vi "myBOT-Simulate-2DOF-ZV.vi"() -> ()   [LabVIEW 2013]
doc: "\"myBOT-Simulate-2DOF-ZV\": Simulates a myBOT with 2DOF (alpha and gamma) as a state space model. Nonlinear behavior is optional. The myBOT behavior can be simulated with two controller types:\n1) PID-Controller\n2) Model Based Balance Controller\n\nThis VI was created for the myRIO Balancing Robot Project. See https://decibel.ni.com/content/groups/myrio-balancing-robot for more information and example projects."
uses:
  <vilib>/addons/Control Design/_Model Construction/Data Typedefs.llb/CD Variables.ctl
  <vilib>/Simulation/Scripting/Companion Diagram/SimConfigNode/SimParams.ctl
  <vilib>/Simulation/Scripting/Companion Diagram/SimConfigNode/_simSolvers.ctl
  <vilib>/Simulation/Implementation/Shared/SIMSCR Execution Mode.ctl
  <vilib>/Platform/TimedLoop/XDataNode/timing_clust.ctl
  <vilib>/Platform/TimedLoop/XDataNode/nitl_modes.ctl
  <vilib>/Platform/TimedLoop/XDataNode/wakeup.ctl
  <vilib>/Simulation/Param Hierarchy/Typedefs/SIMPH Param Control Actions.ctl
  <vilib>/Simulation/Scripting/Editor Utilities/SIM subVI tag data.ctl
  <vilib>/Simulation/Scripting/Editor Utilities/SIM subVI execution type.ctl
  <vilib>/Simulation/Implementation/Shared/NILVSim_ParamChanged.vi
  <vilib>/Simulation/Implementation/Shared/NILVSim_FinishedLate.vi
  <vilib>/Simulation/Implementation/Shared/NILVSIM_BeginStep.vi
  <vilib>/Simulation/Utility/Implementation/SIM Halt.vi
  <vilib>/Simulation/DataSources/Implementation/NILVSim Pulse Generator.llb/SIM Pulse Generator (scalar).vi
  <vilib>/Simulation/ContinuousLinear/Implementation/NILVSim State Space.llb/SIM State Space Distributor (CD).vi
  <vilib>/Simulation/Nonlinear/Implementation/NILVSim Saturation.llb/SIM Saturation (scalar).vi
  <vilib>/Simulation/Implementation/Shared/SIM Is Init or Final Stage.vi
  <vilib>/Simulation/Nonlinear/Implementation/NILVSim DeadZone.llb/SIM DeadZone (scalar).vi
  <vilib>/Simulation/ContinuousLinear/Implementation/NILVSim State Space.llb/SIM State Space Collector (CD).vi
  <vilib>/Simulation/SignalDisplay/Implementation/NILVSim Time Waveform.llb/SIM Time Waveform (vector).vi
  <vilib>/Simulation/Implementation/Shared/SIM Fire Discrete SubVI.vi
  <vilib>/Simulation/Implementation/Shared/NILVSim_Manager.vi
  <vilib>/Simulation/Implementation/Shared/NILVSim_FinalizeModel.vi
  <vilib>/Simulation/Implementation/Shared/SIM Fire Discrete SubVI (Core).vi
  <vilib>/addons/Control Design/_Model Construction/Model Creation.llb/Model Creation SubVI/cd_Create Symbolic State Space Model.vi
  <vilib>/Simulation/Implementation/Shared/SIM Unbundle Sim Info.vi
  <vilib>/Utility/error.llb/Clear Errors.vi
  <vilib>/Simulation/Implementation/Shared/NILVSim_GetModelError.vi
  <vilib>/Simulation/Implementation/Shared/SIM Bundle Sim Info.vi
  <vilib>/Simulation/Implementation/Shared/SIMSH Read Queue.vi
  <vilib>/Simulation/Implementation/Shared/NILVSim_Initialize.vi
  <vilib>/Simulation/Utility/Implementation/NILVSim Get Time and IsAcceptedStep.vi
  SubVI/myBOT_Draw.vi
  SubVI/myBOT_Nonlinearities.vi
  <vilib>/Simulation/Scripting/Companion Diagram/SimConfigNode/SimDog.xnode
  <vilib>/Simulation/Model Libraries/PID/SIM PID (Parallel).vi
  <vilib>/Simulation/Model Libraries/PID/SIM PID.vi
  <vilib>/Platform/TimedLoop/XDataNode/XDataNode.xnode
  <vilib>/Simulation/Implementation/XNodeFramework/SimXNode/SimX.xnode
  <vilib>/addons/Control Design/_Model Construction/NI_LinSys_Model Creation.lvlib
  <vilib>/addons/Control Design/_Model Construction/Model Typedefs.llb/CD General Elements.ctl
  <vilib>/addons/Control Design/_Model Construction/NI_LinSys_Model Typedefs.lvlib
  <vilib>/addons/Control Design/_Model Construction/Model Typedefs.llb/CD State Space Model (MIMO).ctl
  <vilib>/Simulation/ContinuousLinear/Implementation/NILVSim State Space.llb/SIM State Space (CD).vi
  <vilib>/Platform/TimedLoop/XDataNode/XDNodeRunTimeDep.lvlib
  <vilib>/Simulation/Implementation/Shared/NI_SIM_Implementation.lvlib
  <vilib>/addons/Control Design/_Model Construction/NI_LinSys_Data Typedefs.lvlib
panel:
  in  "Controller:\nBalanceController\nPID":bool=TRUE
  in  "Nonlinearities:\nON\nOFF":bool=TRUE
  in  "Kd":dbl
  in  "Kp":dbl=12.0
  in  "myBOT Physical Parameter":T1=[{"Name"="m", " Value"=0.65}, {"Name"="M", " Value"=0.04}, {"Name"="R", " Value"=0.04}, {"Name"="l", " Value"=0.05}, {"Name"="g", " Value"=9.81}, {"Name"="mu", " Value"=0.05}] {"Value" format="%.2f"}
  in  "Stop":bool
  out "3D Picture Control":refnum<vi>(3d-picture)
  out "Waveform Chart":waveform(dbl)[](graph)=[{"t0"=timestamp(15 s since 1904-01-01), "dt"=1.0, "Y"=[-1.0]}, {"t0"=timestamp(15 s since 1904-01-01), "dt"=1.0, "Y"=[1.69]}, {"t0"=timestamp(15 s since 1904-01-01), "dt"=1.0, "Y"=[-13.575559261946736]}, {"t0"=timestamp(15 s since 1904-01-01), "dt"=1.0, "Y"=[-0.23249999999999998]}, {"t0"=timestamp(15 s since 1904-01-01), "dt"=1.0, "Y"=[13004948.530995548]}, {"t0"=timestamp(15 s since 1904-01-01), "dt"=1.0, "Y"=[-24.467999999258332]}]
  in  "Step Size (s)":dbl=0.005
  in  "Final Time (s)":dbl=15.0
  in  "Initial Time (s)":dbl
  # "Controller Settings"
  # "Simulation Parameters"
  # "Balance Controller"
  # "Kp=12, Kd=-6 works"
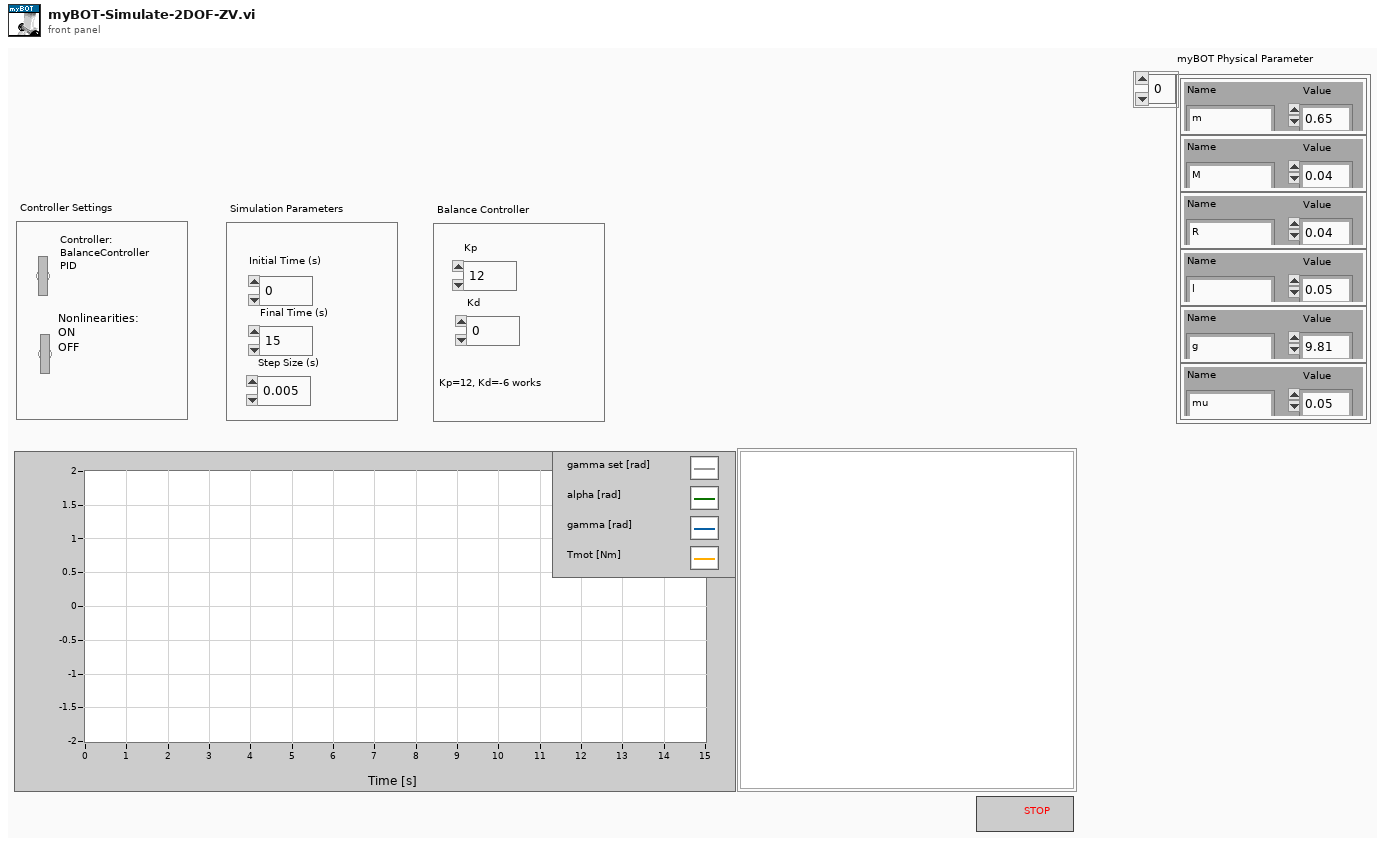
[diagram p1: front panel]
types:
  T1 = typedef "NI_LinSys_Data Typedefs.lvlib/CD Variables.ctl" = cluster{"Name":string, " Value":dbl}[]
  T2 = typedef "NI_LinSys_Model Typedefs.lvlib/CD State Space Model (MIMO).ctl" = cluster{"properties":T3, "A":dbl[][], "B":dbl[][], "C":dbl[][], "D":dbl[][], "StateNames":string[], "Transport Delay":dbl[][]}
  T3 = typedef "NI_LinSys_Model Typedefs.lvlib/CD General Elements.ctl" = cluster{"Model name":string, "Input names":string[], "Output names":string[], "Input Delays":dbl[], "Output Delays":dbl[], "Sampling Time":dbl, "Notes":string}
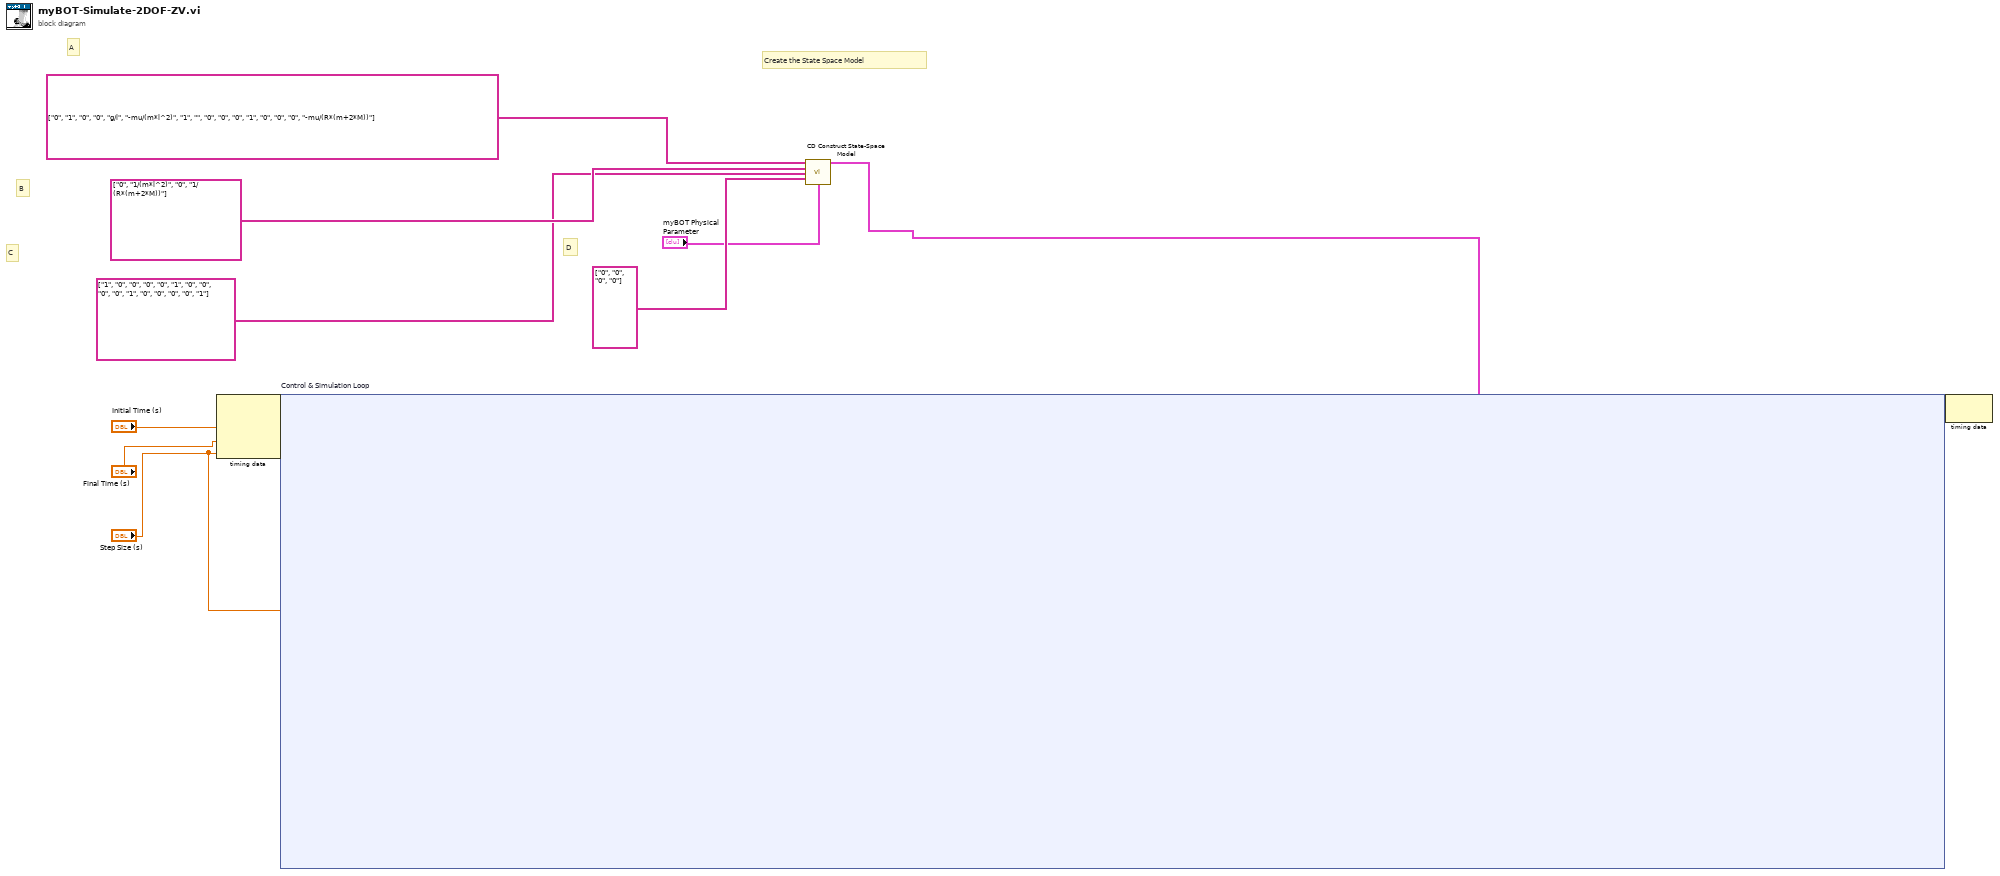
[diagram p0: block diagram]
diagram:
  # "Create the State Space Model"
  # "D"
  # "C"
  # "A"
  # "B"
  n1 = node-c288("Initial Time (s)", "Final Time (s)", "Step Size (s)") -> (w11:variant)  [unwired: 1 in]
  n2 = call-poly <vilib>:"CD Construct State-Space Model.vi"("Symbolic A"=string[][] [["0", "1", "0", "0"], ["g/l", "-mu/(m*l^2)", "1", ""], ["0", "0", "0", "1"], ["0", "0", "0", "-mu/(R*(m+2*M))"]], "Symbolic B"=string[][] [["0"], ["1/(m*l^2)"], ["0"], ["1/(R*(m+2*M))"]], "Symbolic C"=string[][] [["1", "0", "0", "0"], ["0", "1", "0", "0"], ["0", "0", "1", "0"], ["0", "0", "0", "1"]], "Symbolic D"=string[][] [["0"], ["0"], ["0"], ["0"]], "Variables"="myBOT Physical Parameter") -> ("State Space Model"=w1:T2)  [unwired: 9 in, 1 out]
  n3 = node-c254 "Control & Simulation Loop"(w11, w1, "Step Size (s)") -> (w10:variant)
  n4 = node-c288(w10) -> ()  [unwired: 1 out]
